vi "Smooth Interpolation Tool.vi"() -> ()   [LabVIEW 2015, in "RealTimeFilter.lvlib"]
uses:
  RealTimeFilter.lvlib
  TypeDefs/Modes.ctl
  <vilib>/Utility/file.llb/Read Delimited Spreadsheet (DBL).vi
panel:
  in  "Smoothness (1+)":dbl=1.0
  in  "Tab Control":enum32{"Array", "Over time"}(tab)=enum."Over time"
  out "Output":dbl[][](array[numeric])
  out "Input":dbl[][](array[numeric])
  out "Input":dbl[][](graph)
  out "Output":dbl[][](graph)
  in  "Times to multiply":i32=4
  in  "End column":i32=7
  in  "Start column":i32=5
  in  "Start row":i32=1
  in  "Input file":path=path "E:/Data/Dropbox/Documents/Summer2016/Real time filter/9.csv"
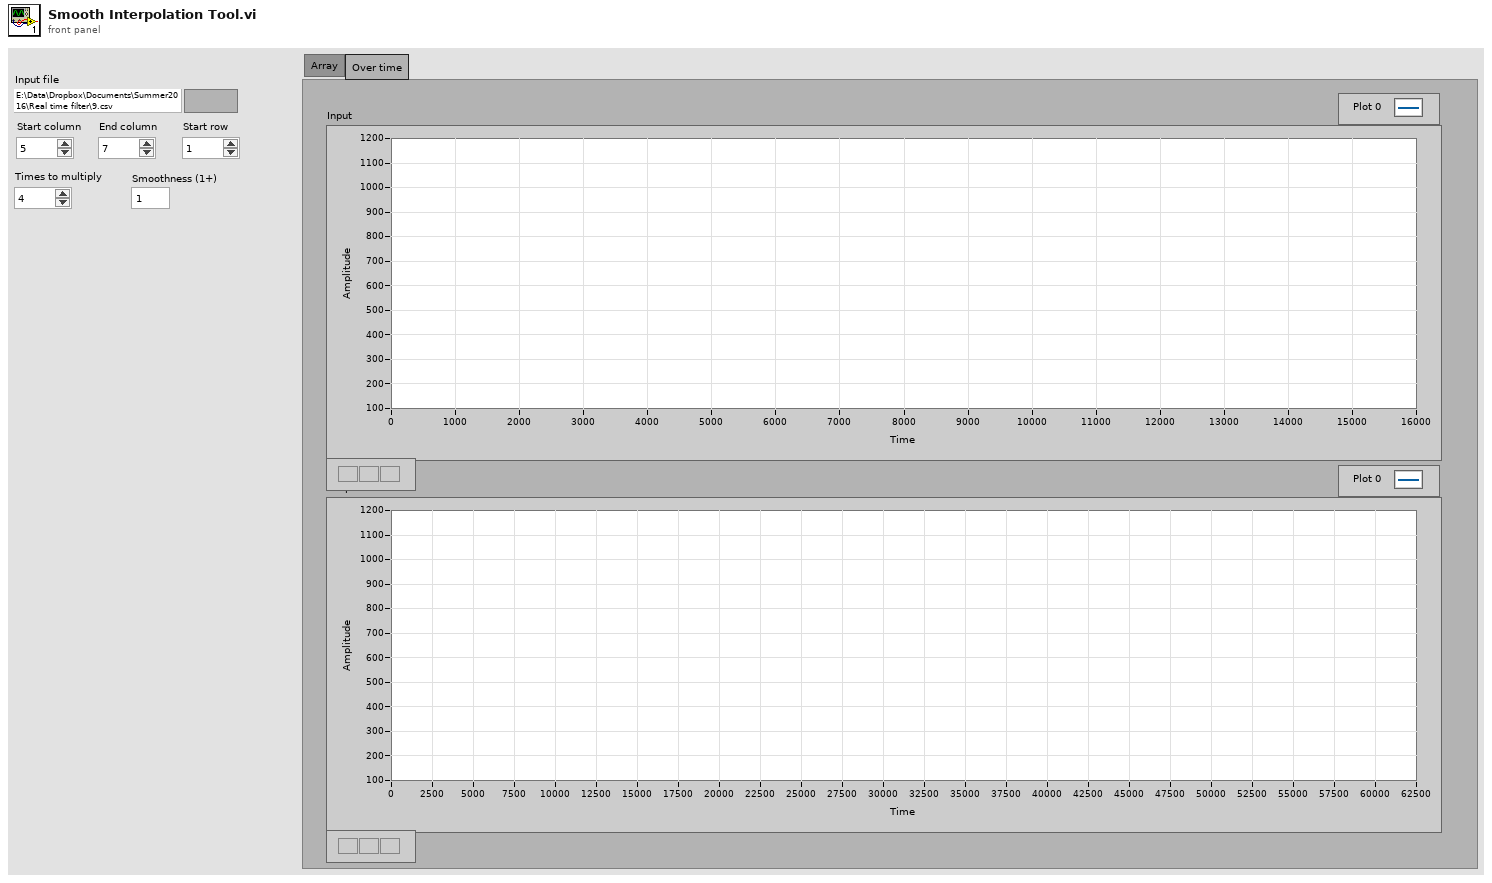
[diagram p1: front panel]
types:
  T1 = typedef "RealTimeFilter.lvlib/Modes.ctl" = enum16{"Sinusoidal", "Gaussian"}
  T2 = typedef "RealTimeFilter.lvlib/Parameters.ctl" = cluster{"number of elements":i32, "start value":dbl, "sinusoidal profile":dbl[], "gaussian profile":dbl[]}
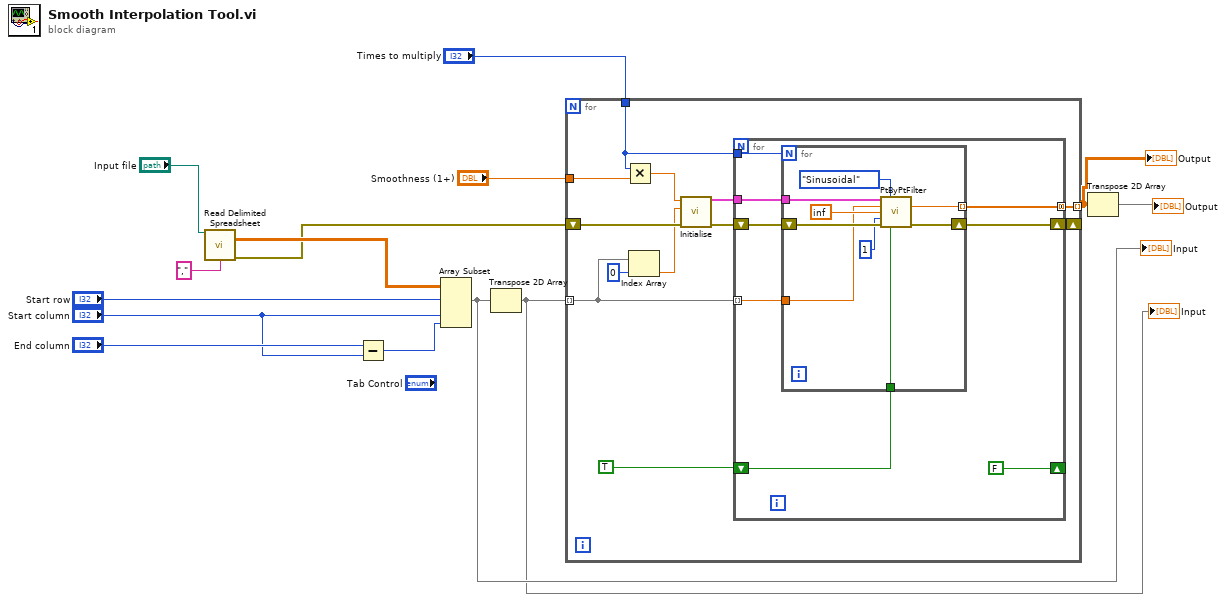
[diagram p0: block diagram]
diagram:
  n1 = call-poly <vilib>:"Read Delimited Spreadsheet.vi"("file path (dialog if empty)"="Input file", "delimiter (\\t)"="," ("delimiter (\\t)")) -> ("all rows"=w12:dbl[][], "error out"=w8:errorcluster)  [unwired: 8 in, 4 out]
  n2 = Subtract(x="End column", y="Start column") -> (x-y=w11:i32)
  n3 = Array Subset(array=w12, index (row)="Start row", index (col)="Start column", length (col)=w11) -> (w4:dbl[][])  [unwired: 1 in]
  "Input" <- w4
  n4 = Transpose 2D Array(2D array=w4) -> (transposed array=w2:dbl[][])
  "Input" <- w2
  n5 = for {
    tunnel: w2 -> [w20] mode=indexing
    shift-right: [w25] -> _
    shift-left: w8 -> [w23]
    tunnel: [w24] -> w3 mode=indexing
    tunnel: "Times to multiply" -> [w17]
    tunnel: "Smoothness (1+)" -> [w15]
    n6 = Multiply(x=w17, y=w15) -> (x*y=w16:dbl)
    n7 = Index Array(array=w20, index=0) -> (element=w18:dbl)
    n8 = call "Initialise.vi"("error in (no error)"=w23, "start value"=w18, "number of elements (max 2048)"=w16) -> ("error out"=w22:errorcluster, "parameter cluster"=w21:T2)  [unwired: 7 in]
    n9 = for {
      tunnel: w20 -> [w30] mode=indexing
      shift-right: [FALSE] -> _
      shift-left: TRUE -> [w29]
      tunnel: w21 -> [w33]
      shift-right: [w31] -> w25
      shift-left: w22 -> [w32]
      tunnel: [w28] -> w24 mode=concatenating
      tunnel: w17 -> [w27]
      n10 = for {
        N: w27 -> [_]
        tunnel: w33 -> [w43]
        shift-right: [w40] -> w31
        shift-left: w32 -> [w41]
        tunnel: w30 -> [w38]
        tunnel: w29 -> [w36]
        tunnel: [w35] -> w28 mode=indexing
        n11 = call "PtByPtFilter.vi"("parameter cluster"=w43, "Mode"=Modes."Sinusoidal", "demand"=w38, "max speed"=inf, "dt"=i64 1, "error in"=w41, "reset"=w36) -> ("filtered signal"=w35:dbl, "error out"=w40:errorcluster)  [unwired: 7 in]
      }
    }
  }
  "Output" <- w3
  n12 = Transpose 2D Array(2D array=w3) -> (transposed array=→"Output":dbl[][])
